vi "start.vi"(0 "HGF_IMAQDevice":refnum<class "HGF_IMAQDevice.lvclass">, 5 "error in (no error)":errorcluster) -> (14 "dup HGF_IMAQDevice":refnum<class "HGF_IMAQDevice.lvclass">, 19 "error out":errorcluster)   [LabVIEW 2014, in "HGF_IMAQ.lvlib" / "HGF_IMAQDevice.lvclass"]
doc: "Starts an asynchronous acquisition that was previously configured with IMAQdx Configure Acquisition.vi. Use IMAQdx Stop Acquisition.vi to stop the acquisition."
uses:
  HGF_IMAQDevice.lvclass
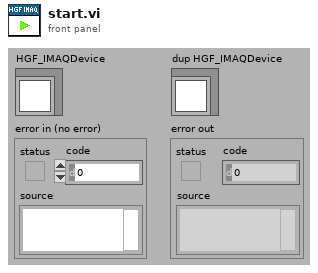
[diagram p1: front panel]
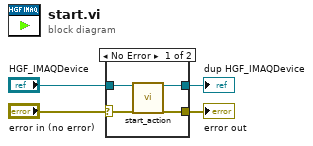
[diagram p0: block diagram]
diagram:
  n1 = case shown="No Error" "error in (no error)" {
    selector: "error in (no error)" -> [w5 w10]
    tunnel: [w6 w10] -> w3
    tunnel: [w7 w9] -> w1
    tunnel: "HGF_IMAQDevice" -> [w8 w9]
    frame No Error {
      n2 = call-dynamic "start_action.vi"("HGF_IMAQDevice"=w8, "error in (no error)"=w5) -> ("dup HGF_IMAQDevice"=w7:refnum<class "HGF_IMAQDevice.lvclass">, "error out"=w6:errorcluster)  [unwired: 16 in]
    }
    frame Error {
    }
  }
  "error out" <- w3
  "dup HGF_IMAQDevice" <- w1
